vi "Mobility-Vt Calculator-File.vi"(5 "Vd_Sat Index":i32, 7 "Vd_Lin Index":i32, 8 "NumPts":i32=5, 9 "Hysteresis Analysis":enum32{"1st Sweep", "2nd Sweep", "Both"}(radio), 10 "Dielectric Constant In":dbl, 11 "Path":path) -> (0 "Used Points":T2, 1 "Graph Cluster":T3, 2 "Vd_Lin":dbl, 3 "Output":T4, 4 "Vd_Sat":dbl)   [LabVIEW 2015]
uses:
  <vilib>/Utility/file.llb/Read From Spreadsheet File (string).vi
panel:
  out "Input Cluster":T1
  out "Off I-Sat":dbl
  out "On/Off I-Sat":dbl
  out "Mobility-Lin":dbl
  out "Vt-Lin":dbl
  out "Vt-Sat":dbl
  out "Mobility-Sat":dbl
  out "Vg Column":dbl[](array[numeric])
  out "Saturation Id":dbl[](array[numeric])
  out "Linear Id":dbl[](array[numeric])
  out "Data Array":string[][](array[string])
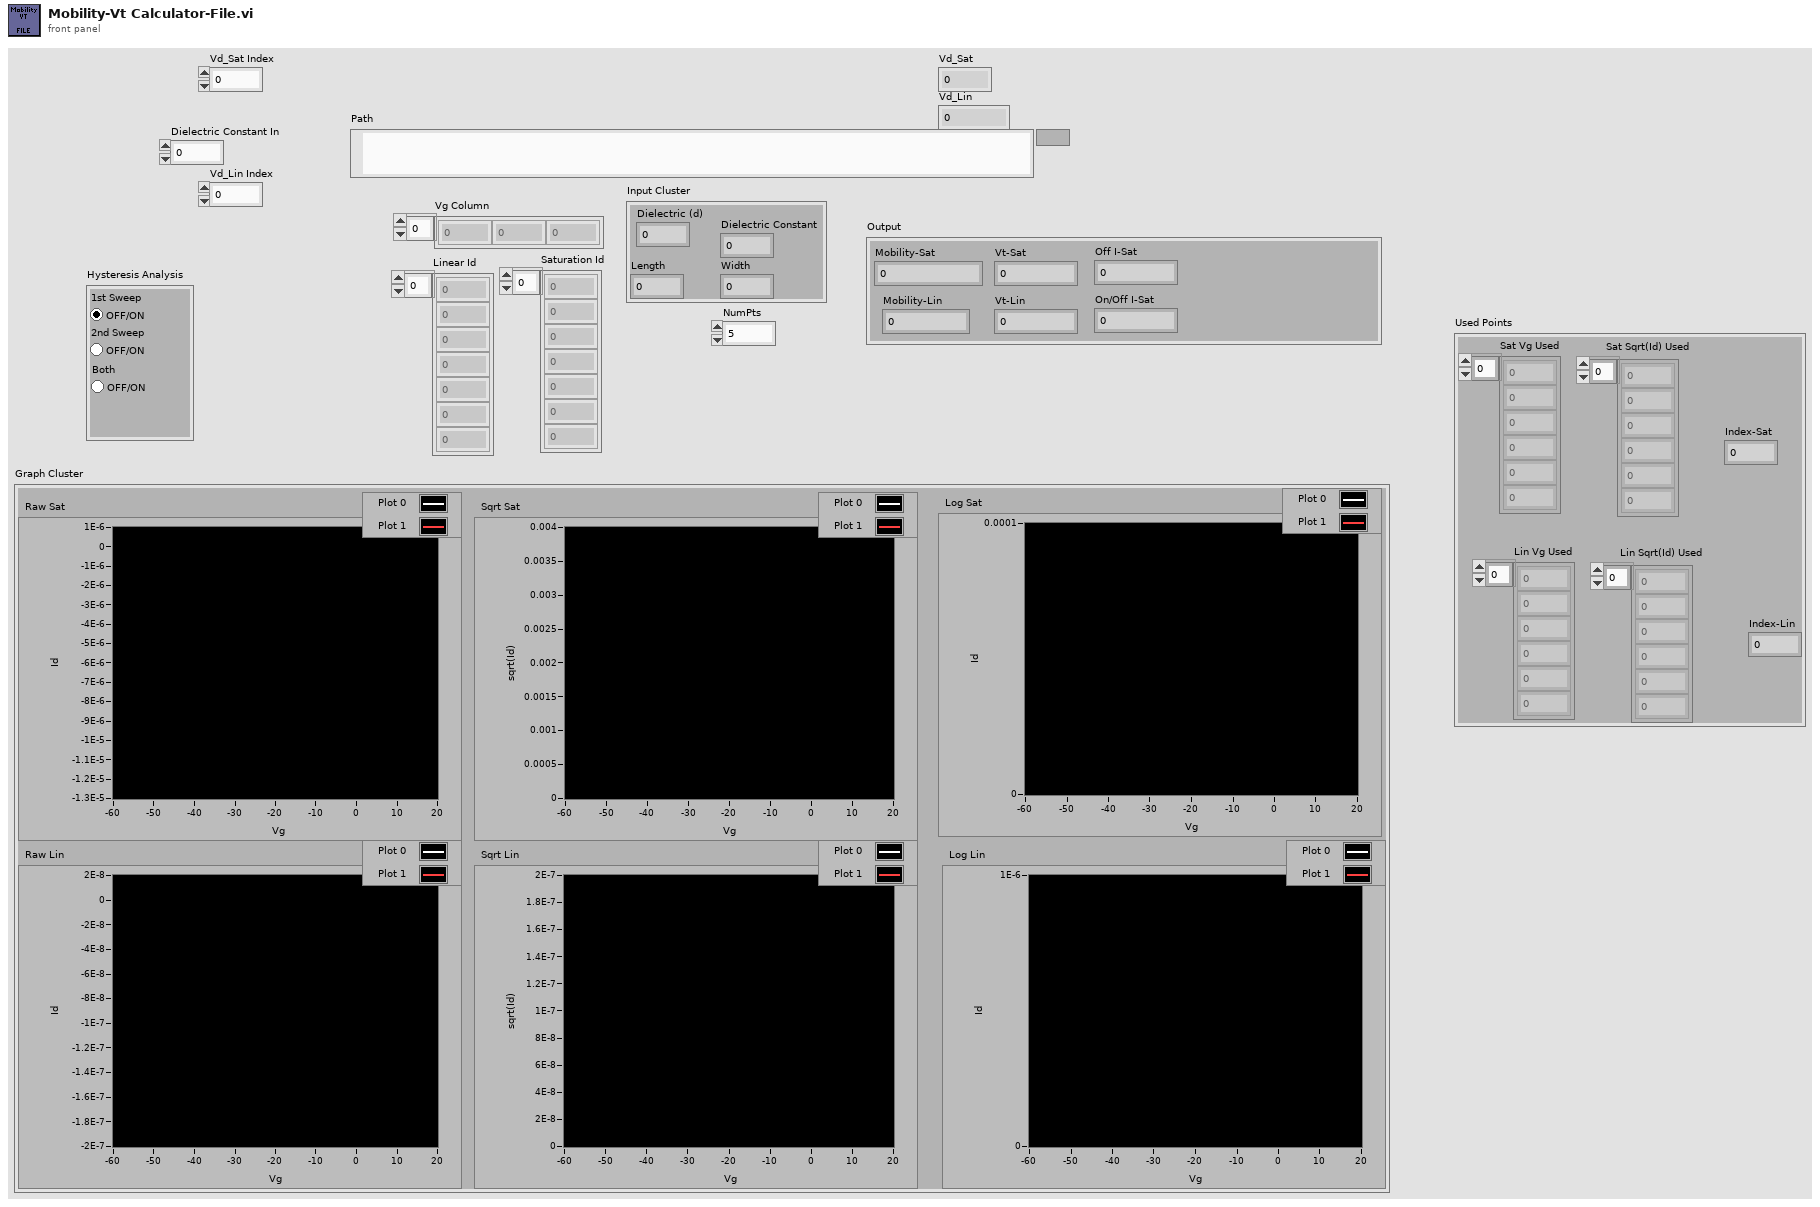
[diagram p1: front panel]
types:
  T1 = cluster{"Length":dbl, "Width":dbl, "Dielectric (d)":dbl, "Dielectric Constant":dbl}
  T2 = cluster{"Sat Vg Used":dbl[], "Sat Sqrt(Id) Used ":dbl[], "Lin Vg Used":dbl[], "Lin Sqrt(Id) Used":dbl[], "Index-Lin":dbl, "Index-Sat":dbl}
  T3 = cluster{"Raw Sat":cluster{dbl[], dbl[]}[], "Sqrt Sat":cluster{dbl[], dbl[]}[], "Log Sat":cluster{dbl[], dbl[]}[], "Raw Lin":cluster{dbl[], dbl[]}[], "Sqrt Lin":cluster{dbl[], dbl[]}[], "Log Lin":cluster{dbl[], dbl[]}[]}
  T4 = cluster{"Mobility-Sat":dbl, "Vt-Sat":dbl, "Mobility-Lin":dbl, "Vt-Lin":dbl, "Off I-Sat":dbl, "On/Off I-Sat":dbl}
  T5 = cluster{"Mobility-Sat":dbl, "VT-Sat":dbl, "Mobility-Lin":dbl, "VT-Lin":dbl, "Off I-Sat":dbl, "On/Off I-Sat":dbl}
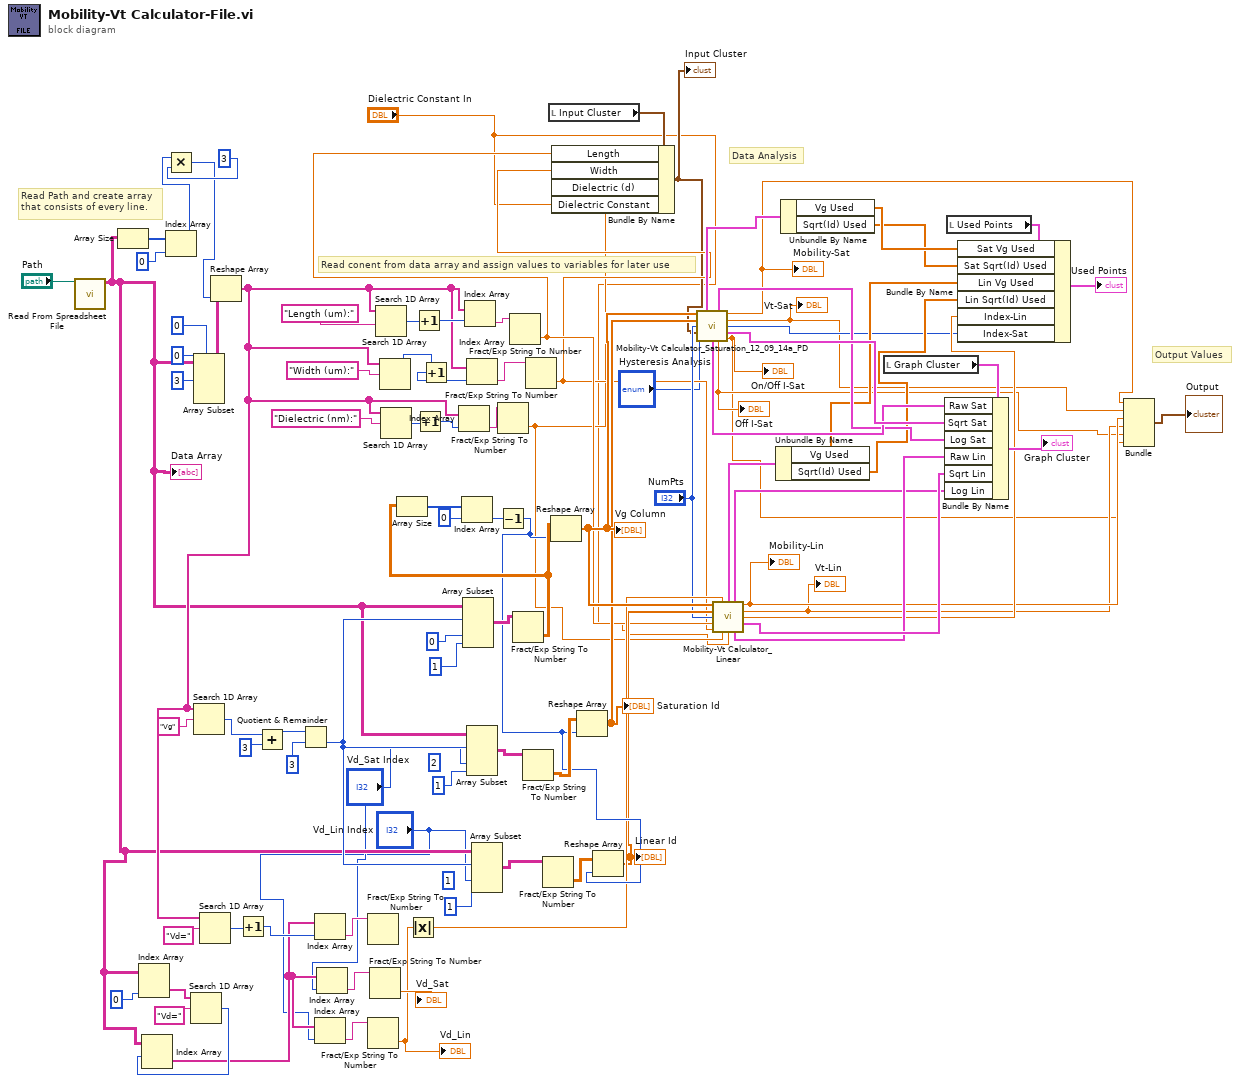
[diagram p0: block diagram]
diagram:
  (unwired) 1
  (unwired) 2
  # "Read Path and create array\nthat consists of every line."
  # "Read conent from data array and assign values to variables for later use"
  # "Data Analysis"
  # "Output Values"
  n1 = call-poly <vilib>:"Read From Spreadsheet File.vi"("file path (dialog if empty)"="Path") -> ("all rows"=w7:string[][])  [unwired: 6 in, 4 out]
  "Data Array" <- w7
  n2 = Array Size(array=w7) -> (size(s)=w77:i32[])
  n3 = Index Array(array=w7, index (col)=0) -> (element=w8:string[])  [unwired: 1 in]
  n4 = Index Array(array=w77, index=0) -> (element=w17:i32)
  n5 = Multiply(x=w17, y=3) -> (x*y=w16:i32)
  n6 = Search 1D Array(1D array=w8, element="Vd=") -> (index of element=w6:i32)  [unwired: 1 in]
  n7 = Index Array(array=w7, index (row)=w6) -> (element=w4:string[])  [unwired: 1 in]
  n8 = Array Subset(array=w7, index (row)=0, index (col)=0, length (col)=3) -> (w72:string[][])  [unwired: 1 in]
  n9 = Reshape Array(w72, w16) -> (w12:string[])
  n10 = Search 1D Array(1D array=w12, element="Vg") -> (index of element=w60:i32)  [unwired: 1 in]
  n11 = Search 1D Array(1D array=w12, element="Vd=") -> (index of element=w11:i32)  [unwired: 1 in]
  n12 = Increment(x=w11) -> (x+1=w41:i32)
  n13 = Add(x=w60, y=3) -> (x+y=w39:i32)
  n14 = Quotient & Remainder(x=w39, y=3) -> (floor(x/y)=w37:i32)  [unwired: 1 out]
  n15 = Index Array(array=w4, index=w41) -> (element=w40:string)
  n16 = Index Array(array=w4, index="Vd_Lin Index") -> (element=w13:string)
  n17 = Index Array(array=w4, index="Vd_Sat Index") -> (element=w15:string)
  n18 = Fract/Exp String To Number(string=w40) -> ()  [unwired: 3 in, 2 out]
  n19 = Fract/Exp String To Number(string=w13) -> (number=w5:dbl)  [unwired: 3 in, 1 out]
  "Vd_Lin" <- w5
  n20 = Fract/Exp String To Number(string=w15) -> (number=→"Vd_Sat":dbl)  [unwired: 3 in, 1 out]
  n21 = Search 1D Array(1D array=w12, element="Length (um):") -> (index of element=w68:i32)  [unwired: 1 in]
  n22 = Search 1D Array(1D array=w12, element="Width (um):") -> (index of element=w69:i32)  [unwired: 1 in]
  n23 = Search 1D Array(1D array=w12, element="Dielectric (nm):") -> (index of element=w64:i32)  [unwired: 1 in]
  n24 = Absolute Value(x=w5) -> (abs(x)=w34:dbl)
  n25 = Increment(x=w68) -> (x+1=w70:i32)
  n26 = Increment(x=w64) -> (x+1=w63:i32)
  n27 = Increment(x=w69) -> (x+1=w71:i32)
  n28 = Index Array(array=w12, index=w63) -> (element=w59:string)
  n29 = Array Subset(array=w7, index (row)=w37, index (col)=0, length (col)=1) -> (w52:string[][])  [unwired: 1 in]
  n30 = Index Array(array=w12, index=w70) -> (element=w57:string)
  n31 = Index Array(array=w12, index=w71) -> (element=w58:string)
  n32 = Array Subset(array=w7, index (row)=w37, index (col)="Vd_Sat Index", length (col)=1) -> (w51:string[][])  [unwired: 1 in]
  n33 = Array Subset(array=w7, index (row)=w37, index (col)="Vd_Lin Index", length (col)=1) -> (w43:string[][])  [unwired: 1 in]
  n34 = Fract/Exp String To Number(string=w59) -> (number=w22:dbl)  [unwired: 3 in, 1 out]
  n35 = Fract/Exp String To Number(string=w57) -> (number=w24:dbl)  [unwired: 3 in, 1 out]
  n36 = Fract/Exp String To Number(string=w52) -> (number=w47:dbl[][])  [unwired: 3 in, 1 out]
  n37 = Array Size(array=w47) -> (size(s)=w48:i32[])
  n38 = Index Array(array=w48, index=0) -> (element=w50:i32)
  n39 = Decrement(x=w50) -> (x-1=w44:i32)
  n40 = Fract/Exp String To Number(string=w51) -> (number=w46:dbl[][])  [unwired: 3 in, 1 out]
  n41 = Fract/Exp String To Number(string=w58) -> (number=w23:dbl)  [unwired: 3 in, 1 out]
  n42 = Fract/Exp String To Number(string=w43) -> (number=w45:dbl[][])  [unwired: 3 in, 1 out]
  n43 = local read "Input Cluster"() -> (w20:T1)
  n44 = Reshape Array(w47, w44) -> (w36:dbl[])
  "Vg Column" <- w36
  n45 = Bundle By Name(cluster=w20, "Length"=w24, "Width"=w23, "Dielectric (d)"=w22, "Dielectric Constant"="Dielectric Constant In") -> (w21:T1)
  "Input Cluster" <- w21
  n46 = Reshape Array(w46, w44) -> (w35:dbl[])
  "Saturation Id" <- w35
  n47 = Reshape Array(w45, w44) -> (w33:dbl[])
  "Linear Id" <- w33
  n48 = call "Mobility-Vt Calculator_Saturation_12_09_14a_PD.vi"("Vg Column"=w36, "Sat Id Column"=w35, "NumPts"="NumPts", "Input Cluster"=w21, "Hysteresis Analysis"="Hysteresis Analysis") -> ("Used Points"=w85:cluster{"Vg Used":dbl[], "Sqrt(Id) Used ":dbl[]}, "Log Graph"=w89:cluster{dbl[], dbl[]}[], "Mobility-Sat"=w29:dbl, "VT-Sat"=w30:dbl, "Index-Sat"=w78:i32, "Sqrt Plot"=w94:cluster{dbl[], dbl[]}[], "Raw Graph"=w93:cluster{dbl[], dbl[]}[], "Off I-Sat"=w26:dbl, "On/Off I-Sat"=w25:dbl)  [unwired: 1 in, 1 out]
  "Vt-Sat" <- w30
  "Mobility-Sat" <- w29
  "Off I-Sat" <- w26
  "On/Off I-Sat" <- w25
  n49 = call "Mobility-Vt Calculator_Linear.vi"("Vg Column"=w36, "Vd"=w34, "Lin Id Column"=w33, "NumPts"="NumPts", "Length"=w24, "Width"=w23, "Dielectric Thickness"=w22, "Dielectric Constant"="Dielectric Constant In") -> ("Used Points"=w82:cluster{"Vg Used":dbl[], "Sqrt(Id) Used ":dbl[]}, "Lin Log"=w90:cluster{dbl[], dbl[]}[], "Mobility-Lin"=w28:dbl, "VT-Lin"=w27:dbl, "Index-Lin"=w79:dbl, "Lin Plot"=w92:cluster{dbl[], dbl[]}[], "Raw Graph"=w91:cluster{dbl[], dbl[]}[])  [unwired: 1 in]
  "Mobility-Lin" <- w28
  "Vt-Lin" <- w27
  n50 = Unbundle By Name(w82) -> ("Vg Used"=w81:dbl[], "Sqrt(Id) Used"=w80:dbl[])
  n51 = Unbundle By Name(w85) -> ("Vg Used"=w84:dbl[], "Sqrt(Id) Used"=w83:dbl[])
  n52 = local read "Graph Cluster"() -> (w95:T3)
  n53 = Bundle By Name(cluster=w95, "Raw Sat"=w93, "Sqrt Sat"=w94, "Log Sat"=w89, "Raw Lin"=w91, "Sqrt Lin"=w92, "Log Lin"=w90) -> (→"Graph Cluster":T3)
  n54 = local read "Used Points"() -> (w87:T2)
  n55 = Bundle By Name(cluster=w87, "Sat Vg Used"=w84, "Sat Sqrt(Id) Used"=w83, "Lin Vg Used"=w81, "Lin Sqrt(Id) Used"=w80, "Index-Lin"=w79, "Index-Sat"=w78) -> (→"Used Points":T2)
  n56 = Bundle("Mobility-Sat"=w29, "VT-Sat"=w30, "Mobility-Lin"=w28, "VT-Lin"=w27, "Off I-Sat"=w26, "On/Off I-Sat"=w25) -> (→"Output":T5)  [unwired: 1 in]
